vi "Update Waveform.vi"(8 "error in (no error)":errorcluster, 11 "Composite Waveform in":refnum<class "Composite Waveform.lvclass">) -> (0 "error out":errorcluster, 3 "Composite Waveform out":refnum<class "Composite Waveform.lvclass">)   [LabVIEW 2014, in "Composite Waveform.lvclass"]
uses:
  Composite Waveform.lvclass
  Composite Waveform.lvclass/Composite Waveform.ctl
  Waveform/Waveform.lvclass/Waveform.ctl
  <vilib>/Waveform/WDTOps.llb/WDT Append Waveforms DBL.vi
  Waveform/Waveform.lvclass
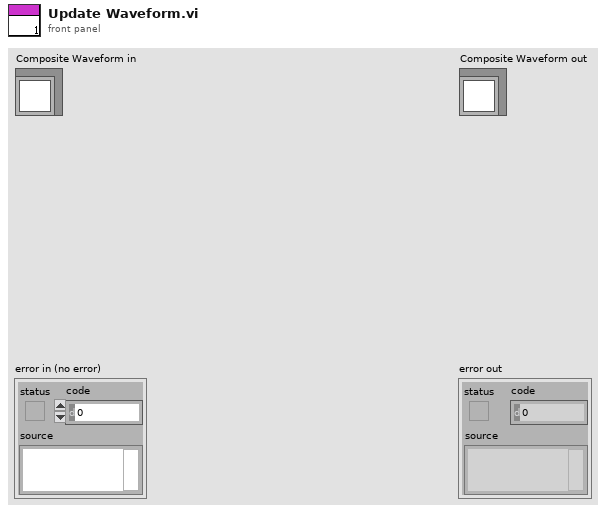
[diagram p1: front panel]
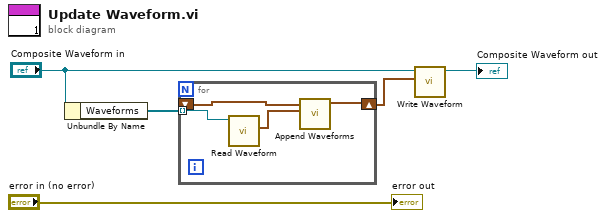
[diagram p0: block diagram]
diagram:
  n1 = Unbundle By Name("Composite Waveform in") -> ("Waveforms"=w3:refnum<class "Waveform.lvclass">[])
  n2 = for {
    tunnel: w3 -> [w9] mode=indexing
    shift-right: [w7] -> w1
    shift-left: _ -> [w6]
    n3 = call "Read Waveform.vi"("Waveform in"=w9) -> ("Waveform"=w8:waveform(dbl))  [unwired: 8 in, 2 out]
    n4 = call-poly <vilib>:"Append Waveforms.vi"("waveform B"=w8, "waveform A"=w6) -> ("waveform out"=w7:waveform(dbl))  [unwired: 8 in, 1 out]
  }
  n5 = call "Write Waveform.vi"("Waveform"=w1, "Waveform in"="Composite Waveform in") -> ("Waveform out"=→"Composite Waveform out":refnum<class "Composite Waveform.lvclass">)  [unwired: 8 in, 1 out]
  "error out" <- "error in (no error)"
